vi "Function Generator.vi"() -> ()   [LabVIEW 2011]
panel:
  in  "Numeric":u32
  out "XY Graph":cluster{"Y":dbl[], "Y":dbl[]}[](graph)
  in  "Divisions \"N\"":dbl=10000.0
  in  "Upper limit \"b\"":dbl=4.2
  in  "Lower limit \"a\"":dbl
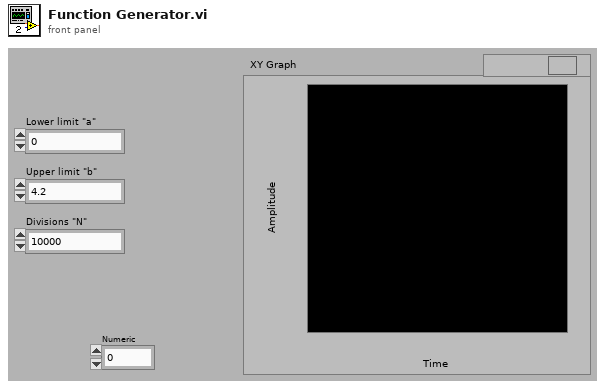
[diagram p1: front panel]
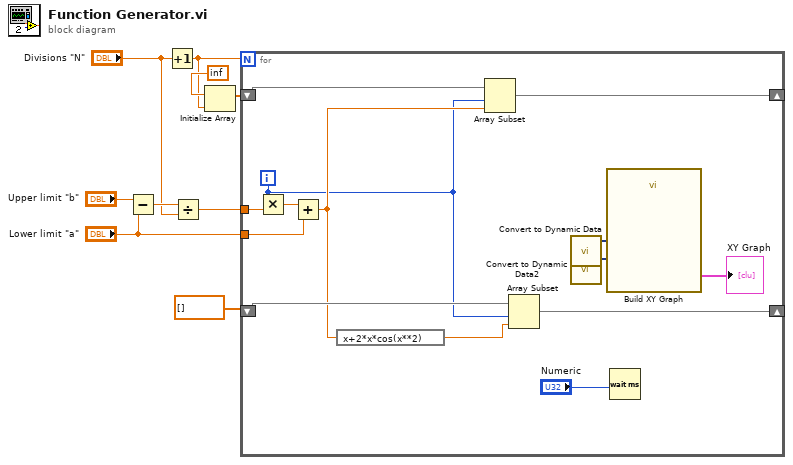
[diagram p0: block diagram]
diagram:
  n1 = Subtract(x="Upper limit \"b\"", y="Lower limit \"a\"") -> (x-y=w8:dbl)
  n2 = Increment(x="Divisions \"N\"") -> (x+1=w1:dbl)
  n3 = Divide(x=w8, y="Divisions \"N\"") -> (x/y=w5:dbl)
  n4 = Initialize Array(inf, w1) -> (w3:dbl[])
  n5 = for {
    N: w1 -> [_]
    tunnel: w5 -> [w23]
    tunnel: "Lower limit \"a\"" -> [w21]
    shift-right: [w16] -> _
    shift-left: w3 -> [w17]
    shift-right: [w14] -> _
    shift-left: dbl[] [] -> [w15]
    i -> [w11]
    n6 = Multiply(x=w11, y=w23) -> (x*y=w22:dbl)
    n7 = Add(x=w22, y=w21) -> (x+y=w12:dbl)
    n8 = expression code="x+2*x*cos(x**2)"(w12) -> (w10:dbl)
    n9 = Array Subset(array=w17, index=w11, length=w12) -> (w16:dbl[])
    n10 = Array Subset(array=w15, index=w11, length=w10) -> (w14:dbl[])
    n11 = call "Convert to Dynamic Data"() -> ("Dynamic Data Type"=w19:dynamicdata)  [unwired: 4 in]
    n12 = call "Convert to Dynamic Data2"() -> ("Dynamic Data Type"=w20:dynamicdata)  [unwired: 4 in]
    n13 = call "Build XY Graph"("Y Input"=w20, "X Input"=w19) -> ("XY Graph"=→"XY Graph":cluster{"Y":dbl[], "Y":dbl[]}[])  [unwired: 3 in, 6 out]
    n14 = Wait (ms)(milliseconds to wait="Numeric") -> ()  [unwired: 1 out]
  }
